vi "BT-sub.vi"(0 "VISA resource name":refnum<visa-resource-name>="COM13", 1 "send data":string, 5 "error in (no error)":errorcluster, 6 "End Write on Termination Character?":bool, 7 "timeout (10sec)":u32=10000, 8 "VISA buffer":i32, 9 "data存盘":bool=TRUE, 10 "mode":T1(ring), 14 "baud rate":u32=57600) -> (15 "timeout?":bool=TRUE, 17 "VISA bytes now":i32, 19 "error IO":errorcluster)   [LabVIEW 2023, in "bt-interface.lvlib"]
uses:
  bt-interface.lvlib
  <vilib>/Instr/_visa.llb/VISA Configure Serial Port (Instr).vi
panel:
  in  "Termination Character":u8=10 format="%.0x"
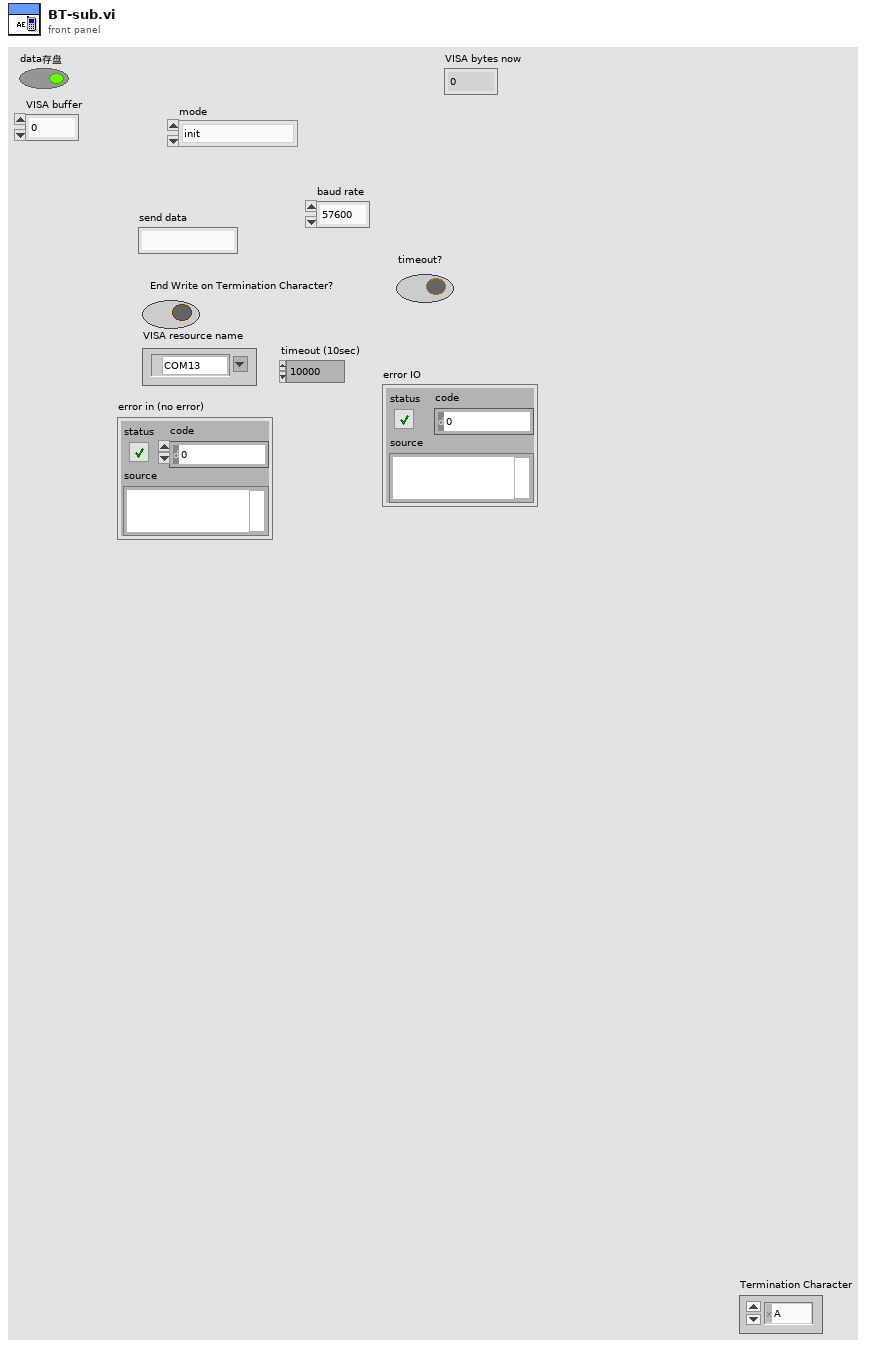
[diagram p1: front panel]
types:
  T1 = enum16{"init", "broadcast_data", "receive_data", "close", "clear_visa"}
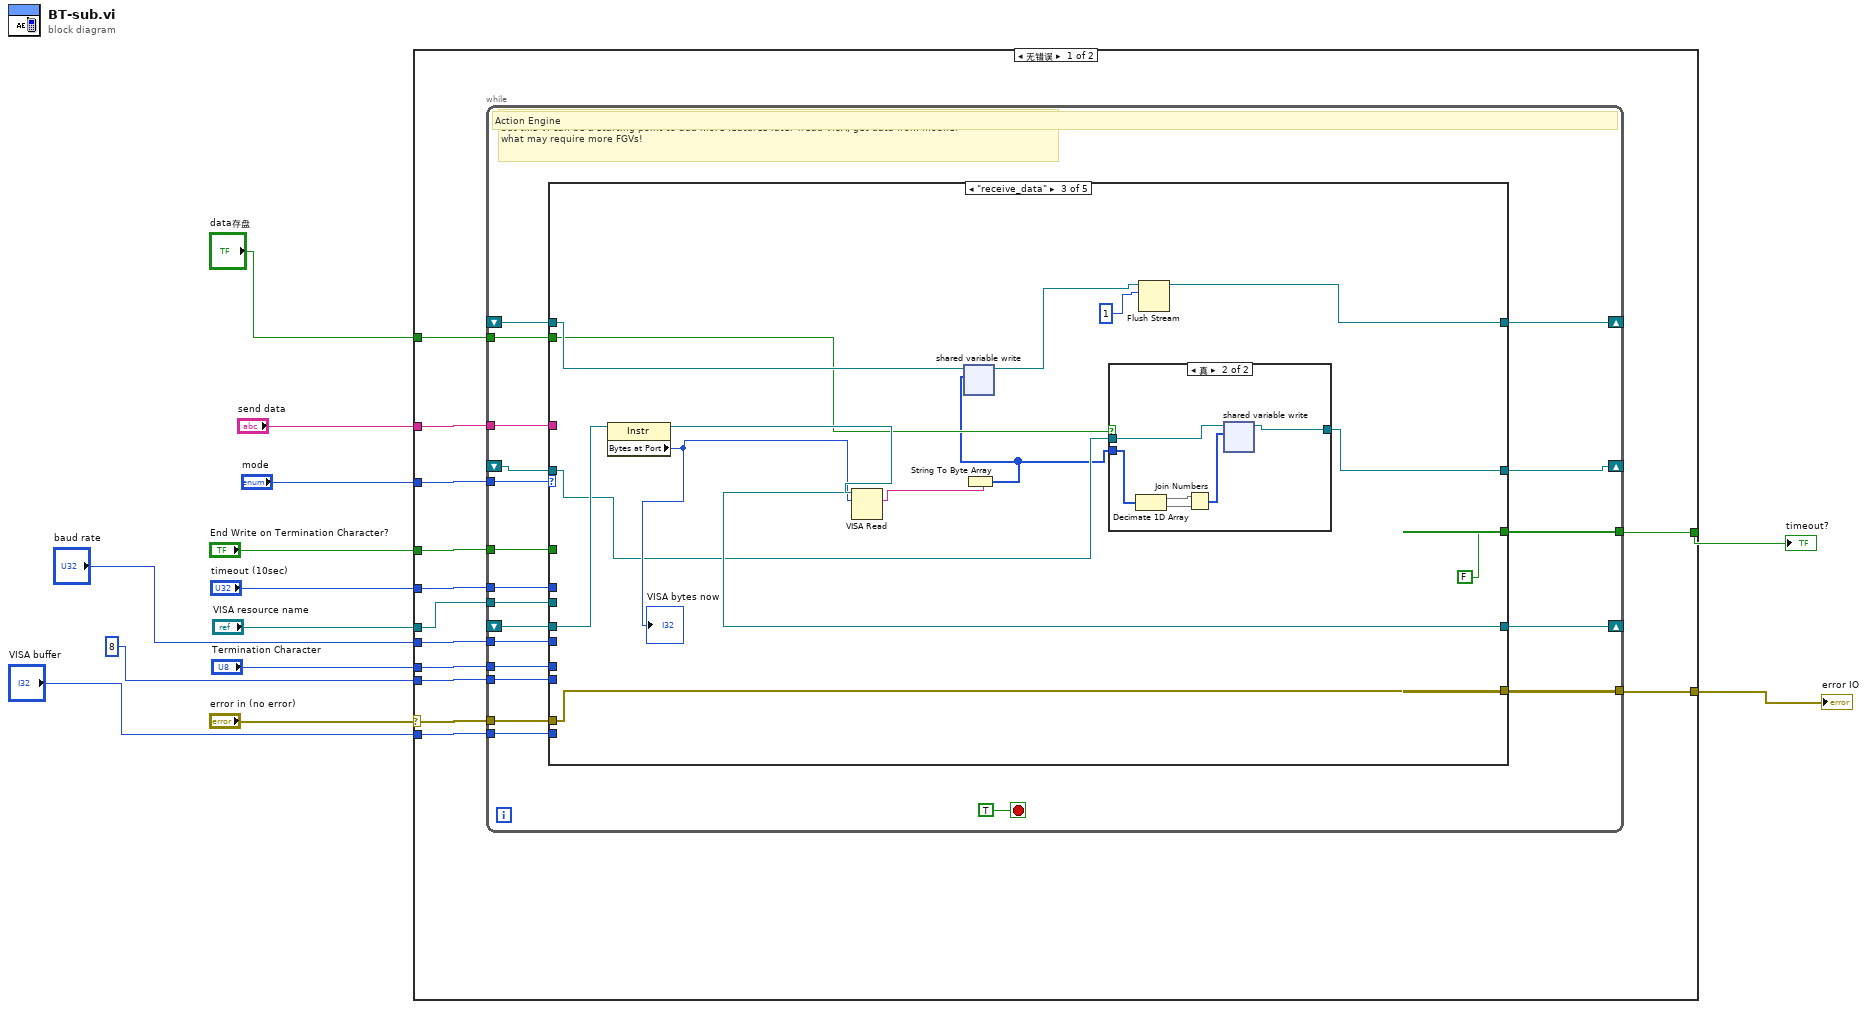
[diagram p0: block diagram]
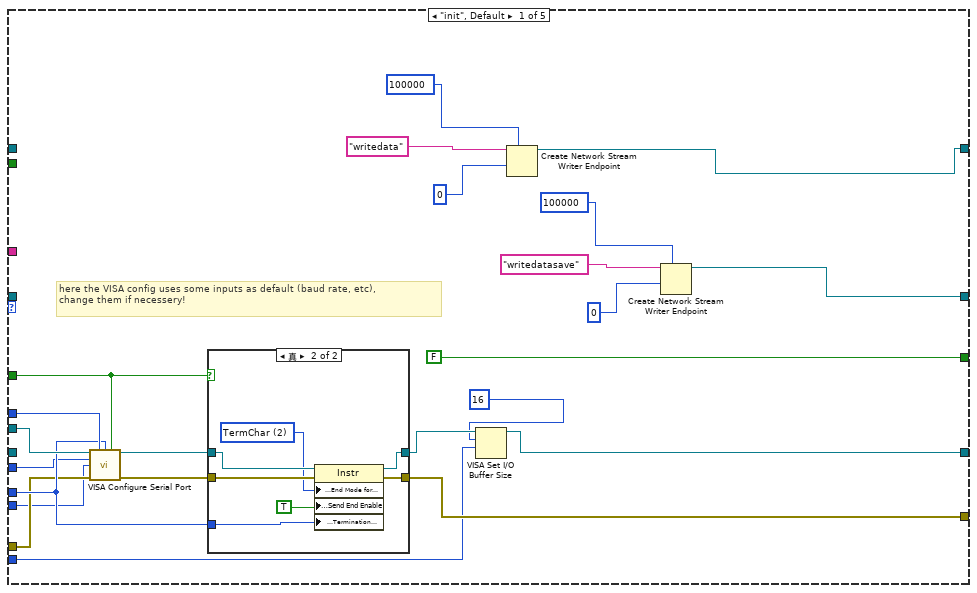
[diagram p2: hidden frame]
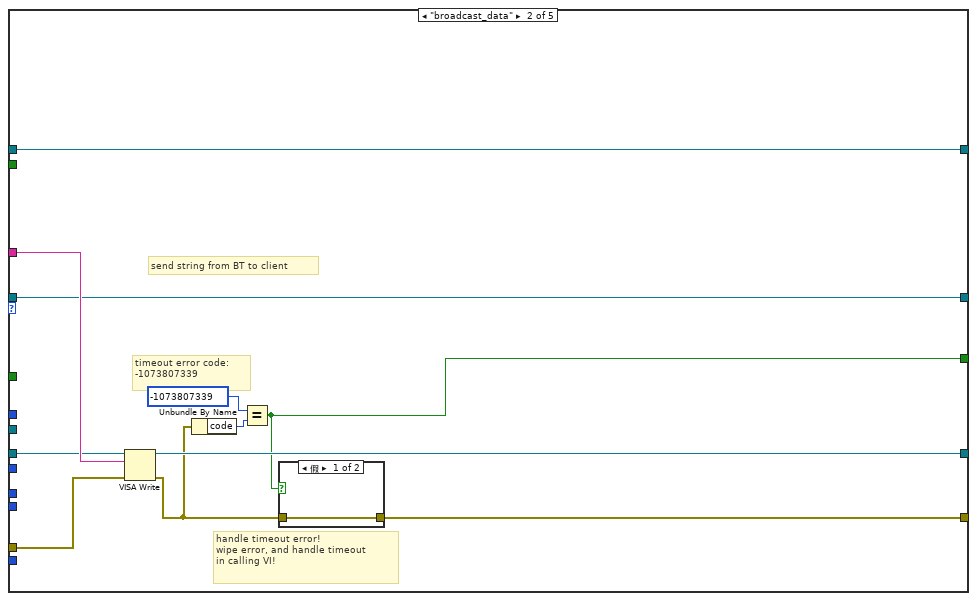
[diagram p4: hidden frame]
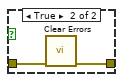
[diagram p5: hidden frame]
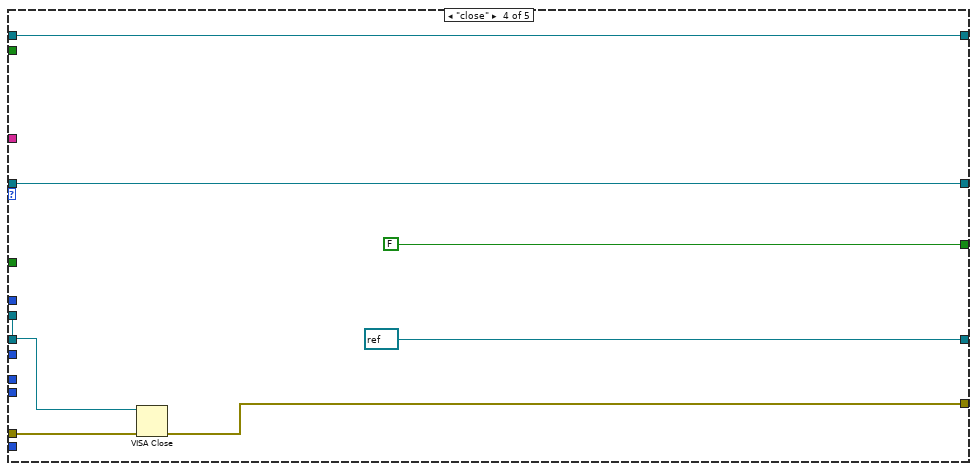
[diagram p7: hidden frame]
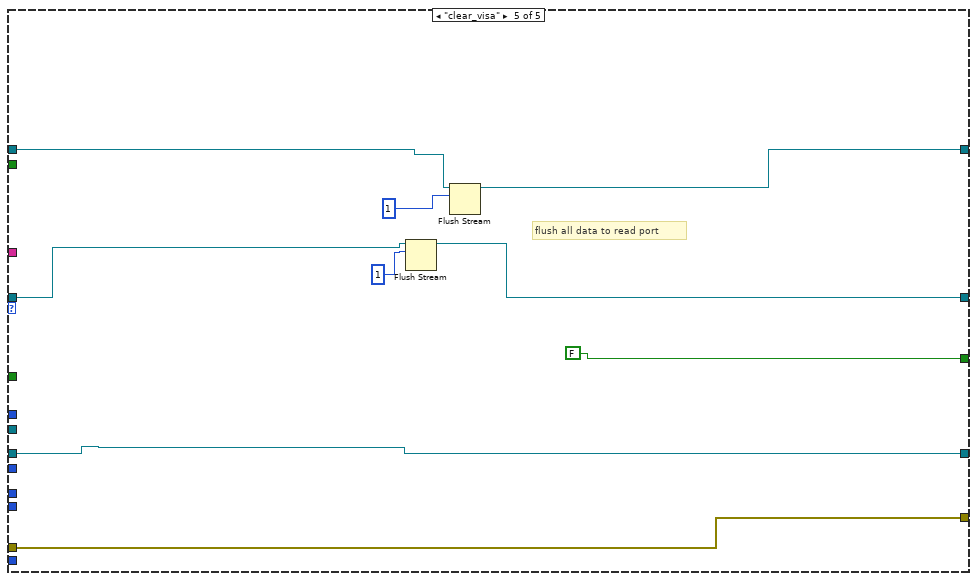
[diagram p8: hidden frame]
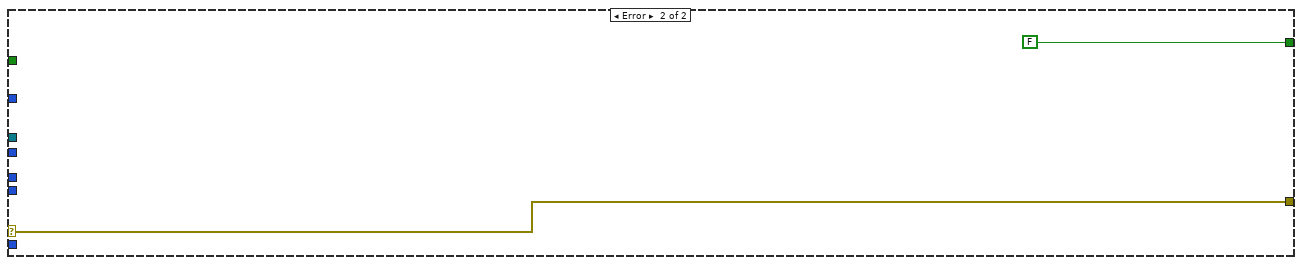
[diagram p9: hidden frame]
diagram:
  n1 = case shown="无错误" "error in (no error)" {
    selector: "error in (no error)" -> [w26 w132]
    tunnel: [w22 w132] -> w12
    tunnel: "mode" -> [w25 _]
    tunnel: "End Write on Termination Character?" -> [w24 _]
    tunnel: "timeout (10sec)" -> [w23 _]
    tunnel: "VISA resource name" -> [w18 _]
    tunnel: "Termination Character" -> [w21 _]
    tunnel: "send data" -> [w20 _]
    tunnel: [w19 FALSE] -> w5
    tunnel: "baud rate" -> [w17 _]
    tunnel: 8 -> [w16 _]
    tunnel: "VISA buffer" -> [w15 _]
    tunnel: "data存盘" -> [w14 _]
    frame No Error {
      n2 = while {
        tunnel: w26 -> [w45]
        tunnel: w25 -> [w44]
        tunnel: w24 -> [w43]
        tunnel: w23 -> [w42]
        shift-right: [w41] -> _
        shift-left: _ -> [w35]
        tunnel: [w40] -> w22
        tunnel: w21 -> [w39]
        tunnel: w20 -> [w38]
        tunnel: [w37] -> w19
        tunnel: w18 -> [w36]
        tunnel: w17 -> [w34]
        tunnel: w16 -> [w33]
        tunnel: w15 -> [w32]
        shift-right: [w31] -> _
        shift-left: _ -> [w30]
        shift-right: [w29] -> _
        shift-left: _ -> [w28]
        tunnel: w14 -> [w27]
        stop <- TRUE stop-if-true
        # "actually this AE does have only 1 FGV yet, \nbut this VI can be a starting point to add more features later (read VISA, get data from mobile)\nwhat may require more FGVs!"
        # "Action Engine"
        n3 = case shown="\"receive_data\"" w44 {
          tunnel: w45 -> [w63 w89 w104 w121 w129]
          tunnel: w43 -> [w61 _ _ _ _]
          tunnel: w42 -> [w67 _ _ _ _]
          tunnel: w36 -> [w66 _ _ w119 _]
          tunnel: [w57 w88 w102 refnum<visa-resource-name> refnum ("VISA resource name out") w124] -> w41
          tunnel: [w65 w86 w104 w120 w129] -> w40
          tunnel: w39 -> [w64 _ _ _ _]
          tunnel: w38 -> [_ w87 _ _ _]
          tunnel: [FALSE w82 FALSE FALSE FALSE] -> w37
          tunnel: w35 -> [_ w81 w107 _ w124]
          tunnel: w34 -> [w60 _ _ _ _]
          tunnel: w33 -> [w59 _ _ _ _]
          tunnel: w32 -> [w55 _ _ _ _]
          tunnel: [w47 w80 w97 w116 w125] -> w31
          tunnel: w30 -> [_ w80 w98 w116 w126]
          tunnel: [w48 w79 w94 w115 w127] -> w29
          tunnel: w28 -> [_ w79 w100 w115 w128]
          tunnel: w27 -> [_ _ w99 _ _]
          frame "init", Default {
            # "here the VISA config uses some inputs as default (baud rate, etc),\nchange them if necessery!"
            n4 = call-poly "VISA Configure Serial Port"("VISA resource name"=w66, "timeout (10sec)"=w67, "termination char\n(0xA = '\\n' = LF)"=w64, "Enable Termination\nChar (T)"=w61, "baud rate (9600)"=w60, "data bits (8)"=w59, "error in (no error)"=w63) -> ("VISA resource name out"=w68:refnum<visa-resource-name>, "error out"=w69:errorcluster)  [unwired: 3 in, 4 out]
            n5 = case shown="真" w61 {
              tunnel: w68 -> [w70 w78]
              tunnel: w69 -> [w71 w77]
              tunnel: [w70 w76] -> w58
              tunnel: [w71 w75] -> w65
              tunnel: w64 -> [_ w73]
              frame False {
              }
              frame True {
                w74 = u16 2 items=["None", "LastBit", "TermChar", "Break"] ("Serial Settings:Serial End Mode for Writes")
                n6 = property class="Instr"(reference=w78, error in=w77, "Serial Settings:End Mode for Writes"=w74, "Message Based Settings:Send End Enable"=TRUE, "Message Based Settings:Termination Character"=w73) -> (reference out=w76:refnum<visa-resource-name>, error out=w75:errorcluster)
              }
            }
            n7 = VISA Set I/O Buffer Size(VISA resource name=w58, mask (16)=16, size (4096)=w55) -> (VISA resource name out=w57:refnum<visa-resource-name>)  [unwired: 1 in, 1 out]
            n8 = Create Network Stream Writer Endpoint(7:100000, 9:u8 0, 11:"writedata") -> (3:w48:refnum<k21>)  [unwired: 4 in, 1 out]
            n9 = Create Network Stream Writer Endpoint(7:100000, 9:u16 0, 11:"writedatasave") -> (3:w47:refnum<k21>)  [unwired: 4 in, 1 out]
          }
          frame "broadcast_data" {
            # "send string from BT to client"
            # "handle timeout error!\nwipe error, and handle timeout\nin calling VI!"
            # "timeout error code:\n-1073807339"
            n10 = VISA Write(VISA resource name=w81, write buffer=w87, error in (no error)=w89) -> (VISA resource name out=w88:refnum<visa-resource-name>, error out=w85:errorcluster)  [unwired: 1 out]
            n11 = Unbundle By Name(w85) -> ("code"=w84:i32)
            n12 = Equal?(x=-1073807339 ("code"), y=w84) -> (x = y?=w82:bool)
            n13 = case shown="假" w82 {
              tunnel: w85 -> [w90 w92]
              tunnel: [w90 w91] -> w86
              frame False {
              }
              frame True {
                n14 = call <vilib>:"Clear Errors.vi"("error in (no error)"=w92) -> ("error out"=w91:errorcluster)  [unwired: 5 in, 1 out]
              }
            }
          }
          frame "receive_data" {
            n15 = property class="Instr"(reference=w107) -> (reference out=w106:refnum<visa-resource-name>, "Bytes at Port"=w103:u32)  [unwired: 1 in, 1 out]
            "VISA bytes now" <- w103
            n16 = VISA Read(VISA resource name=w106, byte count=w103) -> (VISA resource name out=w102:refnum<visa-resource-name>, read buffer=w101:string)  [unwired: 1 in, 2 out]
            n17 = String To Byte Array(string=w101) -> (unsigned byte array=w96:u8[])
            n18 = shared-variable-write(w100, w96) -> (w95:refnum<k21>)  [unwired: 2 in, 2 out]
            n19 = case shown="真" w99 {
              tunnel: w98 -> [w108 w109]
              tunnel: [w108 w110] -> w97
              tunnel: w96 -> [_ w112]
              frame False {
              }
              frame True {
                n20 = Decimate 1D Array(w112) -> (w113:u8[], w114:u8[])
                n21 = Join Numbers(hi=w113, lo=w114) -> ((hi.lo)=w111:u16[])
                n22 = shared-variable-write(w109, w111) -> (w110:refnum<k21>)  [unwired: 2 in, 2 out]
              }
            }
            n23 = Flush Stream(10:1, 11:w95) -> (3:w94:refnum<k21>)  [unwired: 2 in, 2 out]
          }
          frame "close" {
            n24 = VISA Close(VISA resource name=w119, error in (no error)=w121) -> (error out=w120:errorcluster)
          }
          frame "clear_visa" {
            # "flush all data to read port"
            n25 = Flush Stream(10:1, 11:w126) -> (3:w125:refnum<k21>)  [unwired: 2 in, 2 out]
            n26 = Flush Stream(10:1, 11:w128) -> (3:w127:refnum<k21>)  [unwired: 2 in, 2 out]
          }
        }
      }
    }
    frame Error {
    }
  }
  "error IO" <- w12
  "timeout?" <- w5
